vi "Close - Session Json to Data Add Session Instr State Map.vi"(8 "error in":errorcluster, 11 "json in":string) -> (0 "error out":errorcluster, 3 "data out":T1)   [LabVIEW 2020, in "MeasurementServerTests.lvlib"]
uses:
  MeasurementServerTests.lvlib
  Runtime/MeasurementLink Session Management/Session Reservation/Data.ctl
  Runtime/MeasurementLink Session Management/Connection Map/Connection Map.lvclass
  Runtime/MeasurementLink Session Management/IState/IState.lvclass
  Runtime/MeasurementLink Session Management/Session Reservation/Session and Driver Info.ctl
  Runtime/MeasurementLink Instrument/IInstrument/IInstrument.lvclass
  Runtime/MeasurementLink Session Management Client/RPC Messages/ni_measurementlink_sessionmanagement_v1_SessionInformation.ctl
  Runtime/MeasurementLink Session Management Client/RPC Messages/nidevice_grpc_Session.ctl
  Runtime/MeasurementLink Session Management Client/RPC Messages/ni_measurementlink_sessionmanagement_v1_ChannelMapping.ctl
  Runtime/MeasurementLink Session Management Client/RPC Messages/ni_measurementlink_PinMapContext.ctl
  Runtime/MeasurementLink Session Management/Reserved State/Reserved State.lvclass
  C:/dev/measurementlink-labview/Source/Runtime/MeasurementLink Session Management/IState/IState.lvclass
  2dfce5ba-96f1-4d0e-9517-3e25601897e8.vi
  Helpers/Fake Instrument/Fake Instrument.lvclass
  C:/dev/measurementlink-labview/Source/Runtime/MeasurementLink Instrument/IInstrument/IInstrument.lvclass
  <vilib>/JDP Science/JSONtext/JSON text to Variant.vi
  <vilib>/JDP Science/JSONtext/LVClass Serializer/JSONtext LVClass Serializer.lvclass
  Runtime/MeasurementLink Session Management/Session Reservation/Session Reservation.lvclass
  Runtime/MeasurementLink Session Management Client/MeasurementLink Session Management Client.lvlib
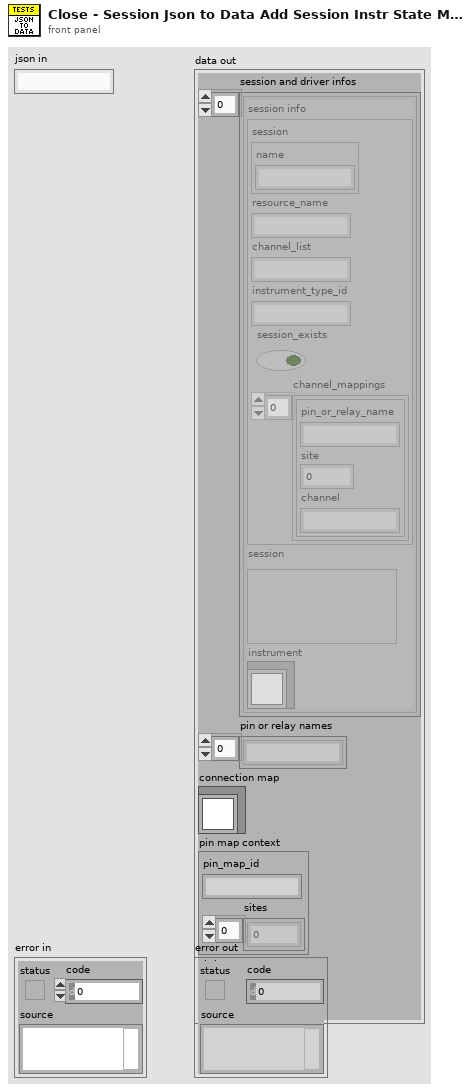
[diagram p1: front panel]
types:
  T1 = typedef "MeasurementLink Session Management.lvlib/Session Reservation.lvclass/Data.ctl" = cluster{"session and driver infos":T2[], "pin or relay names":string[], "connection map":refnum<class "Connection Map.lvclass">, "pin map context":T6, "state":refnum<class "IState.lvclass">}
  T2 = typedef "MeasurementLink Session Management.lvlib/Session Reservation.lvclass/Session and Driver Info.ctl" = cluster{"session info":T3, "session":variant, "instrument":refnum<class "IInstrument.lvclass">}
  T3 = typedef "MeasurementLink Session Management Client.lvlib/ni_measurementlink_sessionmanagement_v1_SessionInformation.ctl" = cluster{"session":T4, "resource_name":string, "channel_list":string, "instrument_type_id":string, "session_exists":bool, "channel_mappings":T5[]}
  T4 = typedef "MeasurementLink Session Management Client.lvlib/nidevice_grpc_Session.ctl" = cluster{"name":string}
  T5 = typedef "MeasurementLink Session Management Client.lvlib/ni_measurementlink_sessionmanagement_v1_ChannelMapping.ctl" = cluster{"pin_or_relay_name":string, "site":i32, "channel":string}
  T6 = typedef "MeasurementLink Session Management Client.lvlib/ni_measurementlink_PinMapContext.ctl" = cluster{"pin_map_id":string, "sites":i32[]}
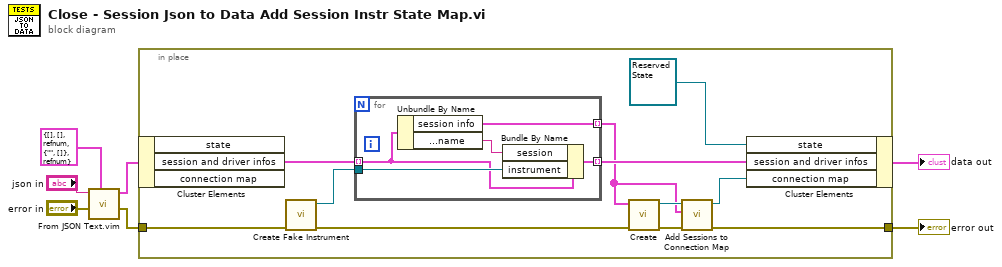
[diagram p0: block diagram]
diagram:
  n1 = call "From JSON Text.vim"("Data Type and Default Value"=T1 {"session and driver infos"=[], "pin or relay names"=[], "connection map"=refnum, "pin map context"={"pin_map_id"="", "sites"=[]}, "state"=refnum} ("data"), "error in (no error)"="error in", "JSON"="json in") -> ("error out"=w2:errorcluster, "Data out"=w5:T1)  [unwired: 7 in]
  n2 = in-place {
    in-place-border: w2 -> [w16]
    in-place-border: [w11] -> w1
    n3 = in-place-cluster #1(w5) -> ("session and driver infos"=w15:T2[])  [unwired: 2 out]
    n4 = call "Create Fake Instrument.vi"("error in"=w16) -> ("error out"=w12:errorcluster, "fake instrument out"=w14:refnum<class "Fake Instrument.lvclass">)  [unwired: 9 in]
    n5 = for {
      tunnel: w15 -> [w19] mode=indexing
      tunnel: w14 -> [w20]
      tunnel: [w22] -> w13 mode=indexing
      tunnel: [w18] -> w8 mode=indexing
      n6 = Unbundle By Name(w19) -> ("session info"=w18:T3, "session info.session.name"=w21:string)
      n7 = Bundle By Name(cluster=w19, "session"=w21, "instrument"=w20) -> (w22:T2)
    }
    n8 = call "Create.vi"("session info"=w8) -> ("connection map"=w10:refnum<class "Connection Map.lvclass">)  [unwired: 10 in]
    n9 = call "Add Sessions to Connection Map.vi"("error in"=w12, "session info"=w8, "connection map in"=w10) -> ("error out"=w11:errorcluster, "connection map out"=w9:refnum<class "Connection Map.lvclass">)  [unwired: 7 in]
    n10 = in-place-cluster #1("state"=refnum<class "Reserved State.lvclass"> refnum ("MeasurementLink Session Management.lvlib:Reserved State.lvclass"), "session and driver infos"=w13, "connection map"=w9) -> (→"data out":T1)
  }
  "error out" <- w1
